vi "Rename Engine to Match Bus.vi"(8 "error in (no error)":errorcluster, 9 "Current Bus Number":i32, 10 "Path to File":string="SPIEngineSOM.vi", 11 "Current Bus Path":path) -> (0 "error out":errorcluster, 3 "New File Path":path)   [LabVIEW 2014, in "Initialization and IO Node Scripting.lvlib"]
uses:
  Initialization and IO Node Scripting.lvlib
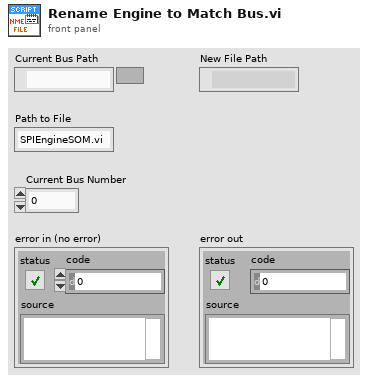
[diagram p1: front panel]
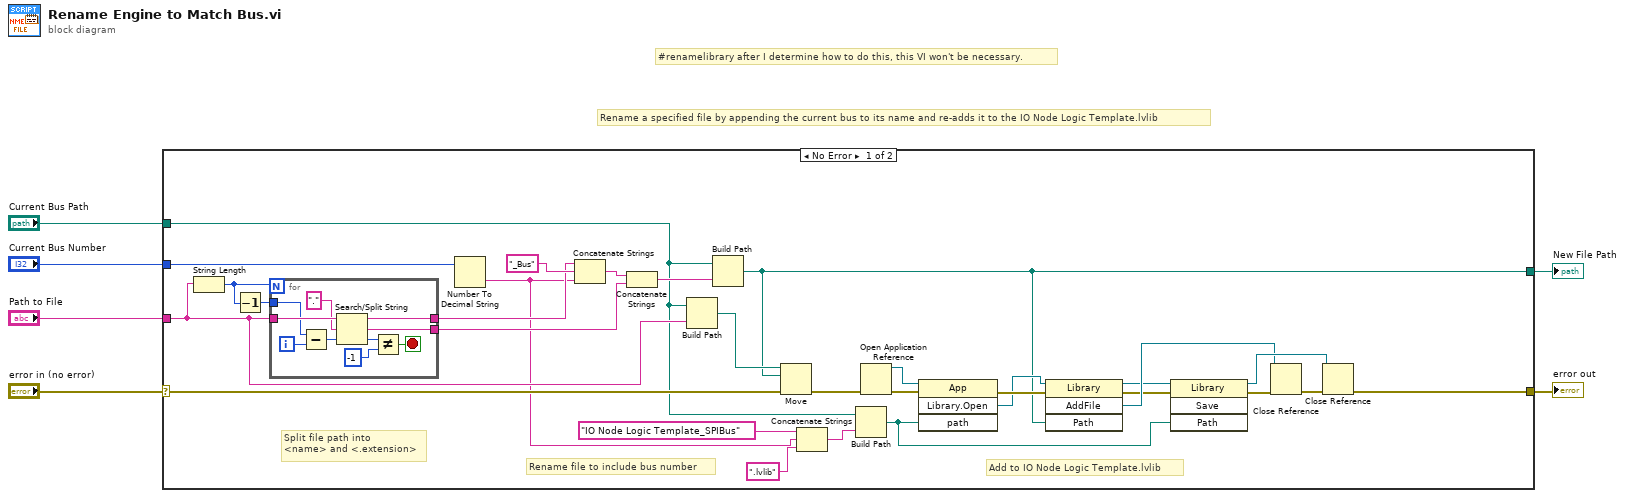
[diagram p0: block diagram]
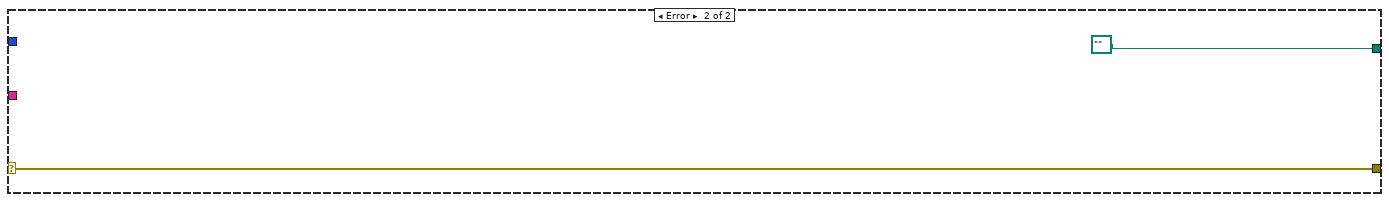
[diagram p2: hidden frame]
diagram:
  # "#renamelibrary after I determine how to do this, this VI won't be necessary."
  # "Rename a specified file by appending the current bus to its name and re-adds it to the IO Node Logic Template.lvlib"
  n1 = case shown="No Error" "error in (no error)" {
    selector: "error in (no error)" -> [w36 w48]
    tunnel: "Current Bus Path" -> [w16 _]
    tunnel: "Current Bus Number" -> [w35 _]
    tunnel: [w26 w48] -> w3
    tunnel: "Path to File" -> [w23 _]
    tunnel: [w9 path "" ("appended path")] -> w1
    frame No Error {
      # "Add to IO Node Logic Template.lvlib"
      # "Split file path into \n<name> and <.extension>"
      # "Rename file to include bus number"
      n2 = String Length(string=w23) -> (length=w25:i32)
      n3 = Decrement(x=w25) -> (x-1=w24:i32)
      n4 = for {
        N: w25 -> [_]
        tunnel: w23 -> [w46]
        tunnel: w24 -> [w41]
        tunnel: [w39] -> w19
        tunnel: [w38] -> w20
        i -> [w40]
        stop <- w43 stop-if-true
        n5 = Subtract(x=w41, y=w40) -> (x-y=w42:i32)
        n6 = Search/Split String(string=w46, search string/char (-)=".", offset (0)=w42) -> (substring before match=w39:string, match + rest of string=w38:string, offset of match=w45:i32)
        n7 = Not Equal?(x=w45, y=-1) -> (x != y?=w43:bool)
      }
      n8 = Number To Decimal String(number=w35) -> (decimal integer string=w17:string)  [unwired: 1 in]
      n9 = Concatenate Strings(w19, "_Bus" ("string"), w17) -> (w22:string)
      n10 = Concatenate Strings(w22, w20) -> (w21:string)
      n11 = Build Path(base path=w16, name or relative path=w23) -> (appended path=w33:path)
      n12 = Build Path(base path=w16, name or relative path=w21) -> (appended path=w9:path)
      n13 = Move(source path=w33, error in=w36, 10:w9) -> (error out=w32:errorcluster)  [unwired: 2 in, 2 out]
      n14 = Concatenate Strings("IO Node Logic Template_SPIBus" ("name or relative path"), w17, ".lvlib" ("string")) -> (w15:string)
      n15 = Build Path(base path=w16, name or relative path=w15) -> (appended path=w11:path)
      n16 = Open Application Reference(8:w32) -> (0:w30:errorcluster, 3:w31:refnum<vi>)  [unwired: 3 in]
      n17 = invoke class="App" method="Library.Open"(reference=w31, error in=w30, "path"=w11) -> (error out=w29:errorcluster, "Open Library"=w28:refnum<vi>)  [unwired: 1 in, 2 out]
      n18 = invoke class="Library" method="AddFile"(reference=w28, error in=w29, "Path"=w9) -> (reference out=w7:refnum<vi>, error out=w8:errorcluster, "AddFile"=w10:refnum<vi>)  [unwired: 1 in, 1 out]
      n19 = invoke class="Library" method="Save"(reference=w7, error in=w8, "Path"=w11) -> (reference out=w13:refnum<vi>, error out=w12:errorcluster)  [unwired: 1 in, 2 out]
      n20 = Close Reference(reference=w10, error in (no error)=w12) -> (error out=w27:errorcluster)
      n21 = Close Reference(reference=w13, error in (no error)=w27) -> (error out=w26:errorcluster)
    }
    frame Error {
    }
  }
  "error out" <- w3
  "New File Path" <- w1
